vi "6812B_AC_cur.vi"() -> ()   [LabVIEW 2019]
doc: "Shows how to generate a standard output."
uses:
  <instrlib>/Agilent 681x Series/Public/Data/Read Single Measurement (Current).vi
  <instrlib>/Agilent 681x Series/Agilent 681x Series.lvlib
panel:
  out "med":bool
  out "Meas":string
  in  "Maximum Time (10000 ms)":i32=10000
  in  "Sense Source (0: Internal)":u16(ring) items=["Internal", "External"]
  in  "Sample Spacing (25 us)":dbl=2.5e-05 format="%^.2g"
  in  "Relative Trigger Samples (0)":i32
  out "Peak Current":dbl
  out "AC + DC RMS Current":dbl
  out "AC RMS Current":dbl
  out "DC Current":dbl
  in  "Pulse Characteristic Value (%)":dbl=50.0 format="%#.4g"
  in  "Pulse Characteristic (0: Duty Cycle)":u16(ring) items=["Duty Cycle", "Pulse Width"]
  in  "Period (s)":dbl=0.03333 format="%#.4g"
  in  "Trigger Delay (s)":dbl format="%#.5g"
  in  "Pulse Count":dbl=1.0 format="%#.4g"
  in  "Voltage Mode (0: Fix)":u16(ring) items=["Fixed", "Step", "Pulse", "List"]
  in  "Triggered Voltage Amplitude (V)":dbl=1.0 format="%#.4g"
  in  "Parar":bool
  in  "Peak Current Limit (13 A)":dbl=13.0 format="%#.4g"
  in  "RMS Current Limit (1 A)":dbl=1.0 format="%#.4g"
  in  "Voltage Amplitude (1.0 V)":dbl=1.0 format="%#.4g"
  in  "Output Frequency (60 Hz)":dbl=60.0 format="%#.4g"
  in  "Output Waveform Type (0: Sinusoid)":u16(ring) items=["Sinusoid", "Square", "Clipped Sinusoid", "User Specified"]
  in  "Serial Configuration":T1={"Baud Rate"=9600, "Parity"=0, "Data Bits"=8} {"Data Bits" items=["7"=7, "8"=8]; "Parity" items=["None", "Odd", "Even", "Mark", "Space"]; "Baud Rate" items=["300"=300, "600"=600, "1200"=1200, "2400"=2400, "4800"=4800, "9600"=9600]}
  in  "VISA resource name":refnum<visa-resource-name>
  # "(c) 2008-2021 National Instruments Corp.  ALL RIGHTS RESERVED."
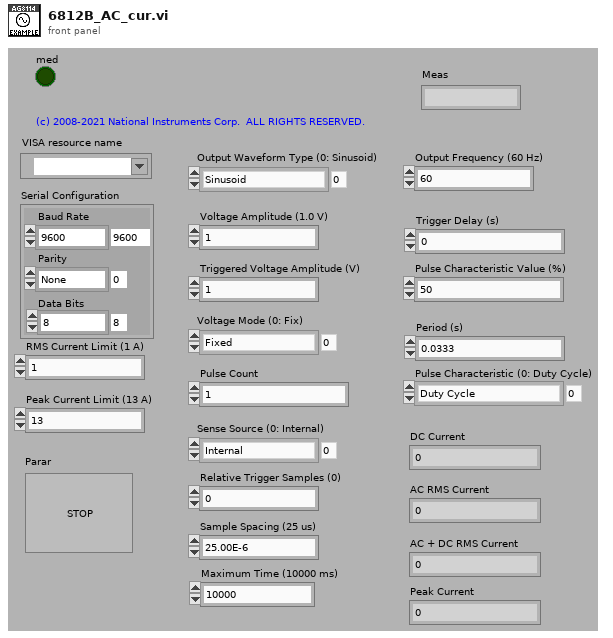
[diagram p1: front panel]
types:
  T1 = cluster{"Baud Rate":u32, "Parity":u16, "Data Bits":u16}
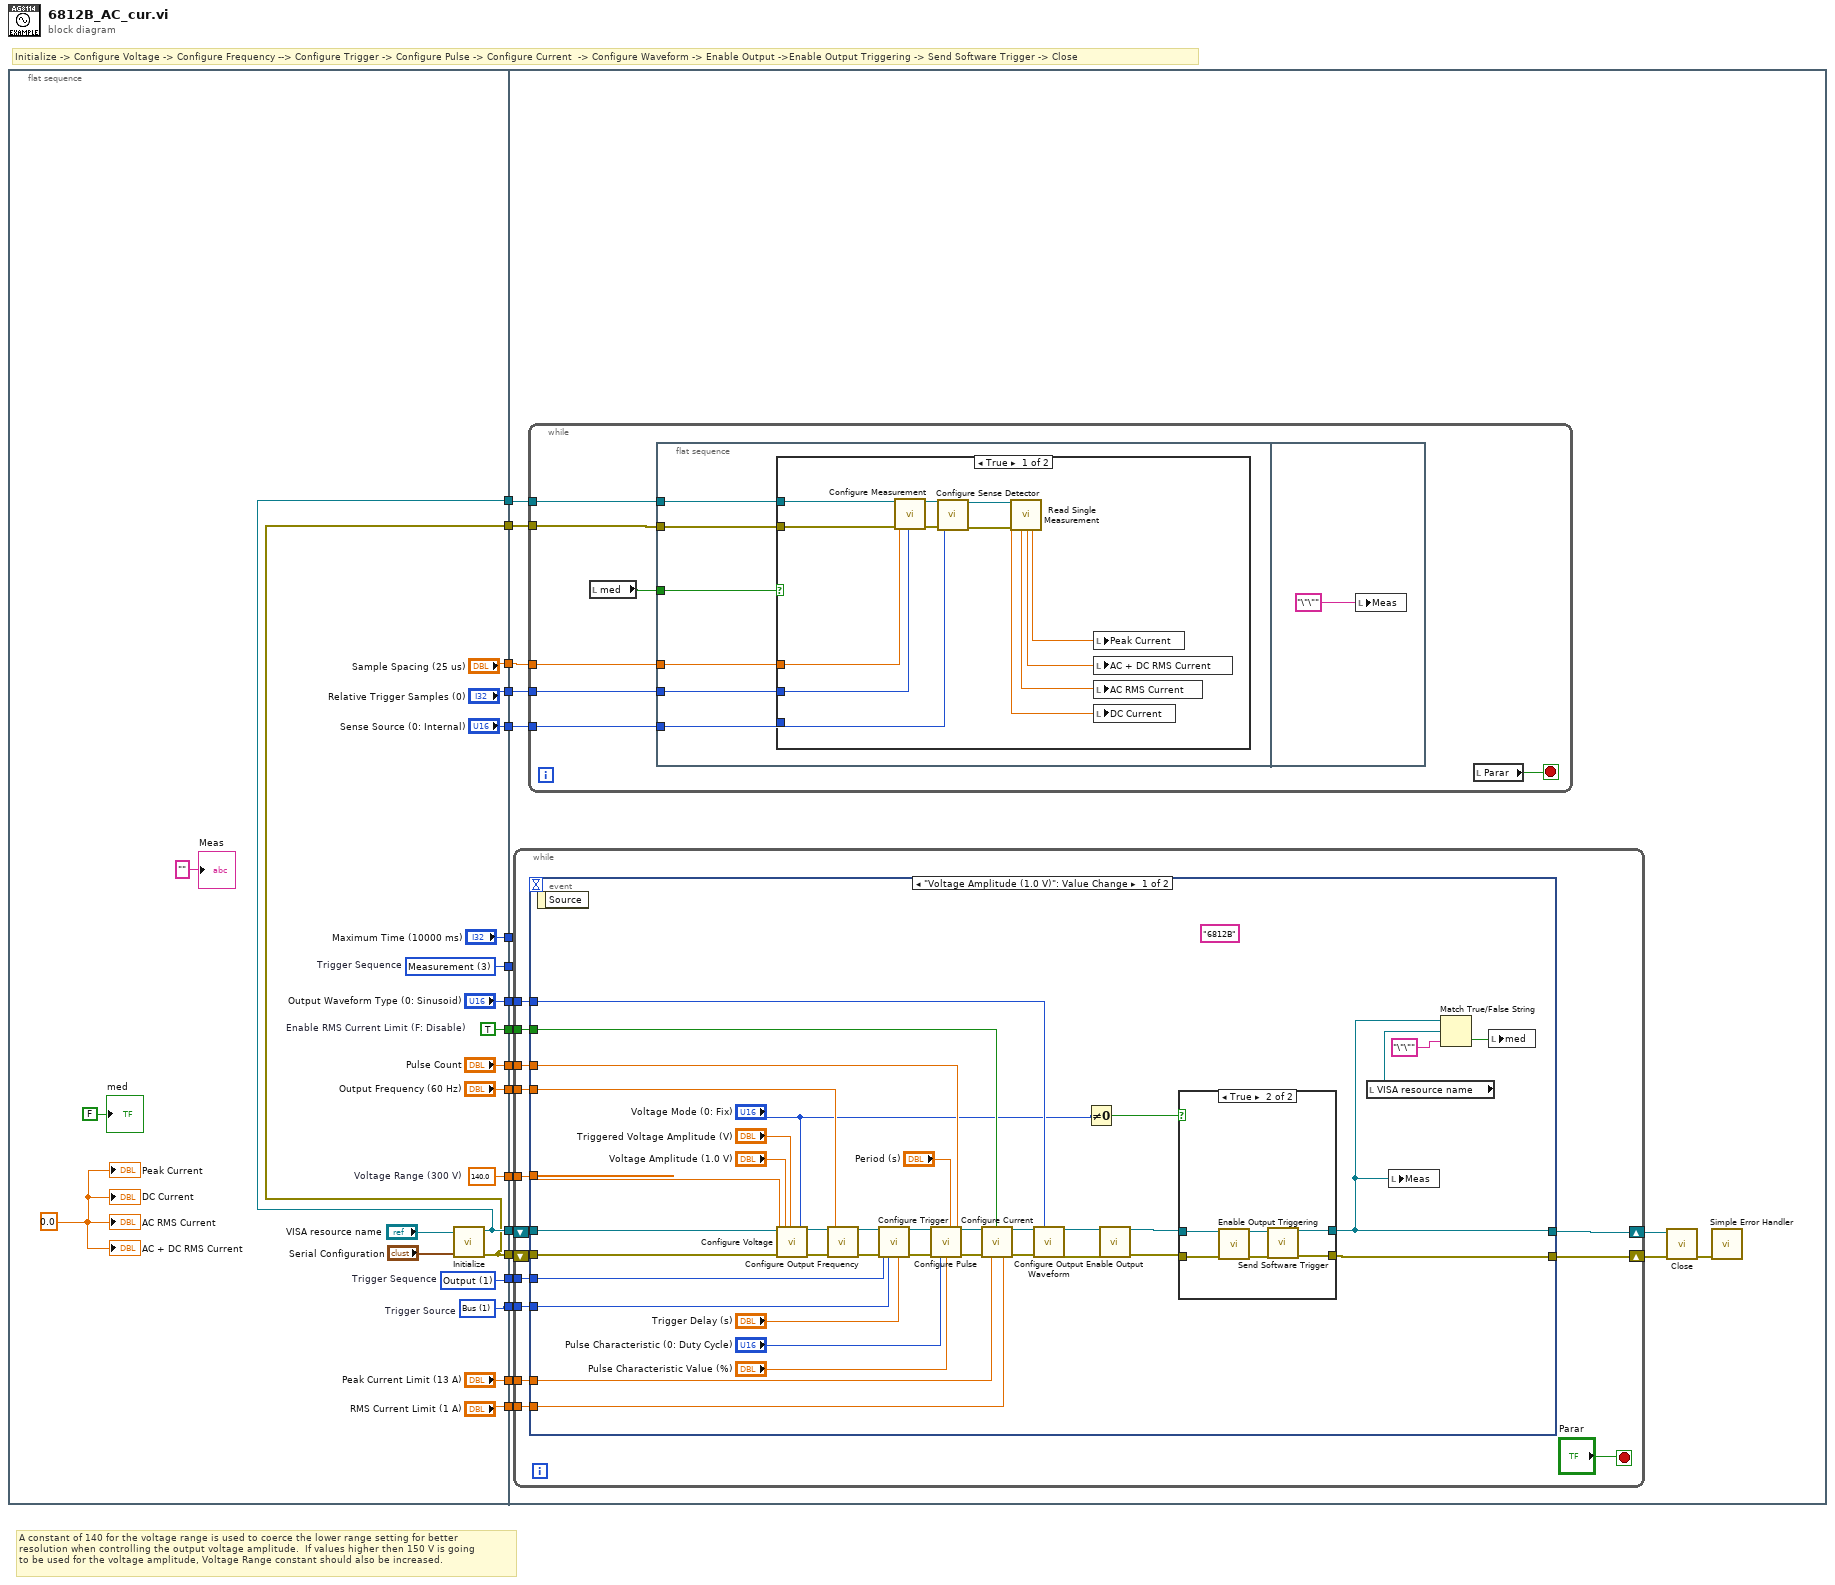
[diagram p0: block diagram]
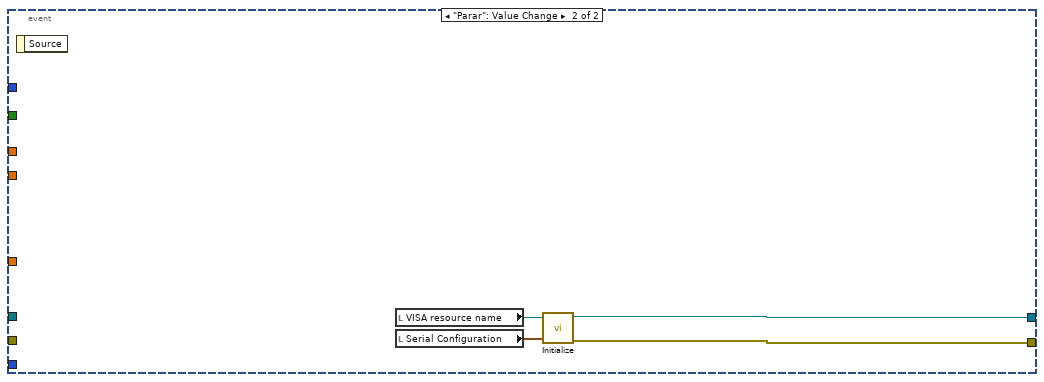
[diagram p4: hidden frame]
diagram:
  # "Initialize -> Configure Voltage -> Configure Frequency --> Configure Trigger -> Configure Pulse -> Configure Current  -> Configure Waveform -> Enable Output ->Enable Output Triggering -> Send Software Trigger -> Close"
  # "A constant of 140 for the voltage range is used to coerce the lower range setting for better\nresolution when controlling the output voltage amplitude.  If values higher then 150 V is going\nto be used for the voltage amplitude, Voltage Range constant should also be increased."
  n1 = flat-sequence {
    tunnel: [w22] -> w18
    tunnel: [w21] -> w17
    tunnel: ["Output Waveform Type (0: Sinusoid)"] -> w16
    tunnel: [w38] -> w15
    tunnel: [w37] -> w14
    tunnel: ["Output Frequency (60 Hz)"] -> w13
    tunnel: ["RMS Current Limit (1 A)"] -> w12
    tunnel: ["Peak Current Limit (13 A)"] -> w11
    tunnel: ["Pulse Count"] -> w10
    tunnel: [w30] -> w9
    tunnel: [w29] -> w8
    tunnel: ["Sense Source (0: Internal)"] -> w7
    tunnel: ["Sample Spacing (25 us)"] -> w6
    tunnel: ["Relative Trigger Samples (0)"] -> w5
    tunnel: [w25] -> w4
    tunnel: ["Maximum Time (10000 ms)"] -> w3
    tunnel: [w22] -> w2
    tunnel: [w21] -> w1
    tunnel: w18 -> [w55]
    tunnel: w17 -> [w45]
    tunnel: w16 -> [w54]
    tunnel: w15 -> [w53]
    tunnel: w14 -> [w52]
    tunnel: w13 -> [w51]
    tunnel: w12 -> [w50]
    tunnel: w11 -> [w49]
    tunnel: w10 -> [w48]
    tunnel: w9 -> [w47]
    tunnel: w8 -> [w46]
    tunnel: w7 -> [w40]
    tunnel: w6 -> [w42]
    tunnel: w5 -> [w41]
    tunnel: w4 -> [_]
    tunnel: w3 -> [_]
    tunnel: w2 -> [w44]
    tunnel: w1 -> [w43]
    frame #0 {
      w23 = 0.0 ("Peak Current")
      w25 = 3 items=["Output"=1, "Synchronous Source"=2, "Measurement"=3]  # Trigger Sequence
      w29 = 1 items=["Immediate", "Bus", "External", "Phase", "Trigger Out"]  # Trigger Source
      w30 = 1 items=["Output"=1, "Synchronous Source"=2, "Measurement"=3]  # Trigger Sequence
      w37 = TRUE  # Enable RMS Current Limit (F: Disable)
      w38 = 140.0  # Voltage Range (300 V)
      n2 = call <instrlib>:"Initialize.vi"("Serial Configuration"="Serial Configuration", "VISA resource name"="VISA resource name") -> ("error out"=w21:errorcluster, "VISA resource name out"=w22:refnum<visa-resource-name>)  [unwired: 8 in]
      "DC Current" <- w23
      "AC RMS Current" <- w23
      "AC + DC RMS Current" <- w23
      "Peak Current" <- w23
      "Meas" <- "" ("Meas")
      "med" <- FALSE ("med")
    }
    frame #1 {
      n3 = while {
        tunnel: w54 -> [w95]
        tunnel: w53 -> [w94]
        tunnel: w52 -> [w93]
        tunnel: w51 -> [w92]
        tunnel: w50 -> [w91]
        tunnel: w49 -> [w90]
        shift-right: [w99] -> w57
        shift-left: w55 -> [w97]
        shift-right: [w98] -> w56
        shift-left: w45 -> [w96]
        tunnel: w48 -> [w89]
        tunnel: w47 -> [w88]
        tunnel: w46 -> [w87]
        stop <- "Parar" stop-if-true
        n4 = event shown="[0] \"Voltage Amplitude (1.0 V)\": Value Change" {
          selector: _ -> [_ _]
          dyn-events: _ -> [_ _]
          timeout: _ -> [_ _]
          tunnel: w97 -> [w113 _]
          tunnel: w96 -> [w112 _]
          tunnel: w95 -> [w137 _]
          tunnel: w94 -> [w136 _]
          tunnel: w93 -> [w135 _]
          tunnel: [w107 w149] -> w98
          tunnel: [w103 w148] -> w99
          tunnel: w92 -> [w129 _]
          tunnel: w91 -> [w134 _]
          tunnel: w90 -> [w133 _]
          tunnel: w89 -> [w120 _]
          tunnel: w88 -> [w116 _]
          tunnel: w87 -> [w110 _]
          event "Voltage Amplitude (1.0 V)": Value Change {
            (unwired) "6812B" ("true string")
            n5 = event-data() -> ()  [unwired: 1 in, 1 out]
            n6 = call <instrlib>:"Configure Voltage.vi"("VISA resource name"=w113, "Triggered Voltage Amplitude (1.0 V)"="Triggered Voltage Amplitude (V)", "Voltage Range (300 V)"=w136, "Voltage Amplitude (1.0 V)"="Voltage Amplitude (1.0 V)", "Voltage Mode (0: Fix)"="Voltage Mode (0: Fix)", "error in (no error)"=w112) -> ("VISA resource name out"=w131:refnum<visa-resource-name>, "error out"=w130:errorcluster)  [unwired: 8 in]
            n7 = call <instrlib>:"Configure Output Frequency.vi"("VISA resource name"=w131, "Output Frequency (60 Hz)"=w129, "error in (no error)"=w130) -> ("VISA resource name out"=w128:refnum<visa-resource-name>, "error out"=w127:errorcluster)  [unwired: 11 in]
            n8 = call <instrlib>:"Configure Trigger.vi"("VISA resource name"=w128, "Trigger Sequence (1: Output 1)"=w116, "Trigger Source (0: Immediate)"=w110, "error in (no error)"=w127, "Trigger Delay (0 s)"="Trigger Delay (s)") -> ("VISA resource name out"=w126:refnum<visa-resource-name>, "error out"=w125:errorcluster)  [unwired: 9 in]
            n9 = call <instrlib>:"Configure Pulse.vi"("VISA resource name"=w126, "Pulse Count (1)"=w120, "Period (0.0333 s)"="Period (s)", "error in (no error)"=w125, "Pulse Characteristic (0: Duty Cycle)"="Pulse Characteristic (0: Duty Cycle)", "Pulse Characteristic Value (50)"="Pulse Characteristic Value (%)") -> ("VISA resource name out"=w124:refnum<visa-resource-name>, "error out"=w123:errorcluster)  [unwired: 8 in]
            n10 = call <instrlib>:"Configure Current.vi"("VISA resource name"=w124, "Enable RMS Current Limit (F: Disable)"=w135, "RMS Current Limit (1 A)"=w134, "error in (no error)"=w123, "Peak Current Limit (13 A)"=w133) -> ("VISA resource name out"=w122:refnum<visa-resource-name>, "error out"=w121:errorcluster)  [unwired: 9 in]
            n11 = call <instrlib>:"Configure Output Waveform.vi"("VISA resource name"=w122, "Output Waveform Type (0: Sinusoid)"=w137, "error in (no error)"=w121) -> ("VISA resource name out"=w108:refnum<visa-resource-name>, "error out"=w109:errorcluster)  [unwired: 11 in]
            n12 = Not Equal To 0?(x="Voltage Mode (0: Fix)") -> (x != 0?=w105:bool)
            n13 = call <instrlib>:"Enable Output.vi"("VISA resource name"=w108, "error in (no error)"=w109) -> ("VISA resource name out"=w104:refnum<visa-resource-name>, "error out"=w106:errorcluster)  [unwired: 12 in]
            n14 = case shown="True" w105 {
              tunnel: w104 -> [w139 w144]
              tunnel: w106 -> [w138 w143]
              tunnel: [w139 w141] -> w103
              tunnel: [w138 w140] -> w107
              frame False {
              }
              frame True {
                n15 = call <instrlib>:"Enable Output Triggering.vi"("VISA resource name"=w144, "error in (no error)"=w143) -> ("VISA resource name out"=w145:refnum<visa-resource-name>, "error out"=w142:errorcluster)  [unwired: 12 in]
                n16 = call <instrlib>:"Send Software Trigger.vi"("VISA resource name"=w145, "error in (no error)"=w142) -> ("VISA resource name out"=w141:refnum<visa-resource-name>, "error out"=w140:errorcluster)  [unwired: 12 in]
              }
            }
            n17 = local read "VISA resource name"() -> (w102:refnum<visa-resource-name>)
            n18 = local write "Meas"(w103) -> ()
            n19 = Match True/False String(2:"\"\"" ("false string"), 3:w102, 4:w103) -> (0:w100:bool)  [unwired: 1 out]
            n20 = local write "med"(w100) -> ()
          }
          event "Parar": Value Change {
            n21 = event-data() -> ()  [unwired: 1 in, 1 out]
            n22 = local read "VISA resource name"() -> (w147:refnum<visa-resource-name>)
            n23 = local read "Serial Configuration"() -> (w146:T1)
            n24 = call <instrlib>:"Initialize.vi"("Serial Configuration"=w146, "VISA resource name"=w147) -> ("error out"=w149:errorcluster, "VISA resource name out"=w148:refnum<visa-resource-name>)  [unwired: 8 in]
          }
        }
      }
      n25 = while {
        tunnel: w44 -> [w65]
        tunnel: w43 -> [w64]
        tunnel: w42 -> [w63]
        tunnel: w41 -> [w62]
        tunnel: w40 -> [w61]
        stop <- w60 stop-if-true
        n26 = local read "med"() -> (w59:bool)
        n27 = flat-sequence {
          tunnel: w65 -> [w71]
          tunnel: w64 -> [w70]
          tunnel: w63 -> [w69]
          tunnel: w62 -> [w68]
          tunnel: w61 -> [w67]
          tunnel: w59 -> [w66]
          frame #0 {
            n28 = case shown="True" w66 {
              tunnel: w71 -> [w84 _]
              tunnel: w70 -> [w83 _]
              tunnel: w69 -> [w82 _]
              tunnel: w68 -> [w81 _]
              tunnel: w67 -> [w80 _]
              frame True {
                n29 = call <instrlib>:"Configure Measurement.vi"("VISA resource name"=w84, "Relative Trigger Samples (0)"=w81, "Sample Spacing (25 us)"=w82, "error in (no error)"=w83) -> ("VISA resource name out"=w78:refnum<visa-resource-name>, "error out"=w79:errorcluster)  [unwired: 10 in]
                n30 = call <instrlib>:"Configure Sense Detector.vi"("VISA resource name"=w78, "Sense Source (0: Internal)"=w80, "error in (no error)"=w79) -> ("VISA resource name out"=w76:refnum<visa-resource-name>, "error out"=w77:errorcluster)  [unwired: 11 in]
                n31 = call-poly <instrlib>:"Read Single Measurement.vi"("VISA resource name"=w76, "error in (no error)"=w77) -> ("Peak Current"=w75:dbl, "DC Current"=w74:dbl, "AC RMS Current"=w73:dbl, "AC + DC RMS Current"=w72:dbl)  [unwired: 8 in, 2 out]
                n32 = local write "Peak Current"(w75) -> ()
                n33 = local write "AC + DC RMS Current"(w74) -> ()
                n34 = local write "AC RMS Current"(w73) -> ()
                n35 = local write "DC Current"(w72) -> ()
              }
              frame False {
              }
            }
          }
          frame #1 {
            n36 = local write "Meas"("\"\"" ("Meas")) -> ()
          }
        }
        n37 = local read "Parar"() -> (w60:bool)
      }
      n38 = call <instrlib>:"Close.vi"("error in (no error)"=w56, "VISA resource name"=w57) -> ("error out"=w58:errorcluster)  [unwired: 9 in]
      n39 = call <vilib>:"Simple Error Handler.vi"("error in (no error)"=w58) -> ()  [unwired: 4 in, 5 out]
    }
  }
